vi "licz srednia.vi"(7 "Array in?":bool, 10 "Waveform in":waveform(dbl), 11 "Array in":dbl[](array[numeric])) -> (3 "Srednia":dbl)   [LabVIEW 2014]
doc: "Liczy wartość średnią z wektora danych"
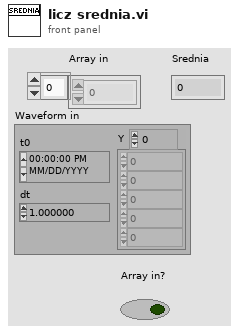
[diagram p1: front panel]
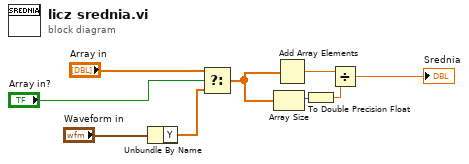
[diagram p0: block diagram]
diagram:
  n1 = Unbundle By Name("Waveform in") -> ("Y"=w4:dbl[])
  n2 = Select(t="Array in", s="Array in?", f=w4) -> (s? t:f=w2:dbl[])
  n3 = Array Size(array=w2) -> (size(s)=w8:i32)
  n4 = Add Array Elements(numeric array=w2) -> (sum=w6:dbl)
  n5 = To Double Precision Float(number=w8) -> (double precision float=w7:dbl)
  n6 = Divide(x=w6, y=w7) -> (x/y=→"Srednia":dbl)
